vi "DB CPLD IOs Channel 2-3.vi"() -> (3 "DBoard IOs":T1)   [LabVIEW 2023]
uses:
  <instrlib>/niUSRP/Reference FPGA/ZBX Control/Dboard IOs.ctl
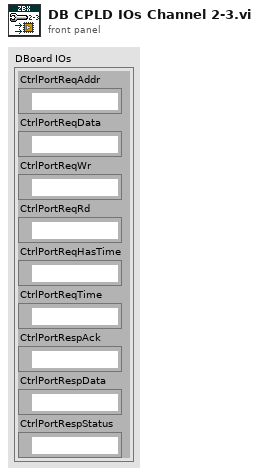
[diagram p1: front panel]
types:
  T1 = typedef "Dboard IOs.ctl" = cluster{"CtrlPortReqAddr":refnum<k21>, "CtrlPortReqData":refnum<k21>, "CtrlPortReqWr":refnum<k21>, "CtrlPortReqRd":refnum<k21>, "CtrlPortReqHasTime":refnum<k21>, "CtrlPortReqTime":refnum<k21>, "CtrlPortRespAck":refnum<k21>, "CtrlPortRespData":refnum<k21>, "CtrlPortRespStatus":refnum<k21>}
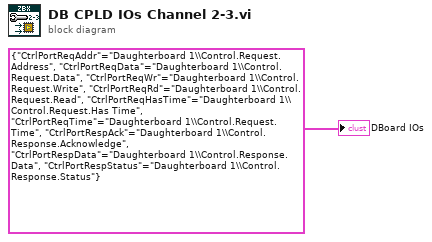
[diagram p0: block diagram]
diagram:
  "DBoard IOs" <- T1 {"CtrlPortReqAddr"="Daughterboard 1\\Control.Request.Address", "CtrlPortReqData"="Daughterboard 1\\Control.Request.Data", "CtrlPortReqWr"="Daughterboard 1\\Control.Request.Write", "CtrlPortReqRd"="Daughterboard 1\\Control.Request.Read", "CtrlPortReqHasTime"="Daughterboard 1\\Control.Request.Has Time", "CtrlPortReqTime"="Daughterboard 1\\Control.Request.Time", "CtrlPortRespAck"="Daughterboard 1\\Control.Response.Acknowledge", "CtrlPortRespData"="Daughterboard 1\\Control.Response.Data", "CtrlPortRespStatus"="Daughterboard 1\\Control.Response.Status"} ("DBoard IOs")
